vi "USS9804_GetDI.vi"(8 "Error In":errorcluster, 11 "Handle":u64) -> (0 "Error Out":errorcluster, 2 "pDI":i32, 3 "Handle 2":u64)   [LabVIEW 2015]
uses:
  USS9804.DLL
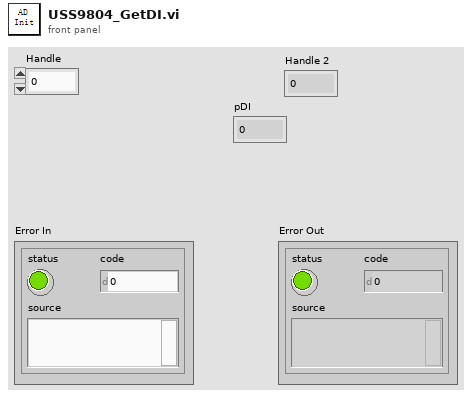
[diagram p1: front panel]
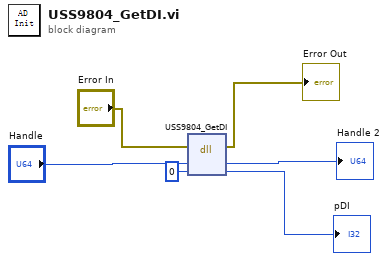
[diagram p0: block diagram]
diagram:
  n1 = dll-call lib="PTH2Sabs CYexinrongWorkplace\t普密斯Thickness-measurementLabVIEWUSS9804.DLL" fn="USS9804_GetDI"(error in="Error In", "Handle"="Handle", "pDI"=0) -> (error out=→"Error Out":errorcluster, "Handle"=→"Handle 2":u64, "pDI"=→"pDI":i32)  [unwired: 3 in, 1 out]
